vi "elapsed_time.vi"(1 "Time since last update":i32, 2 "Initial Time":i32, 3 "Current Time":i32) -> (0 "Elapsed Time":i32)   [LabVIEW 2015]
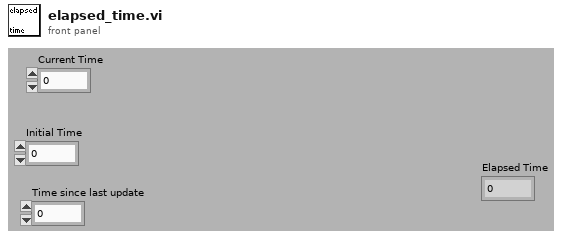
[diagram p1: front panel]
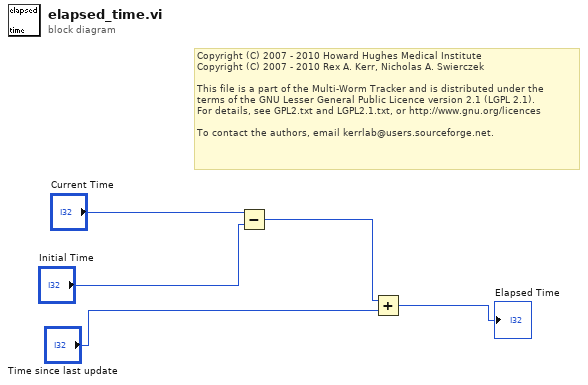
[diagram p0: block diagram]
diagram:
  # "Copyright (C) 2007 - 2010 Howard Hughes Medical Institute\nCopyright (C) 2007 - 2010 Rex A. Kerr, Nicholas A. Swierczek\n \nThis file is a part of the Multi-Worm Tracker and is distributed under the\nterms of the GNU Lesser General Public Licence version 2.1 (LGPL 2.1).\nFor details, see GPL2.txt and LGPL2.1.txt, or http://www.gnu.org/licences\n \nTo contact the authors, email kerrlab@users.sourceforge.net."
  n1 = Subtract(x="Current Time", y="Initial Time") -> (x-y=w5:i32)
  n2 = Add(x=w5, y="Time since last update") -> (x+y=→"Elapsed Time":i32)
